vi "testCustomAssertionFailureMessage.vi"() -> ()   [LabVIEW 2019, in "AssertionTest.lvlib" / "ErrorMessageContainsString.lvlib"]
uses:
  ErrorMessageContainsString.lvlib
  Assertion/Assertion.lvlib
  AssertionTest.lvlib
panel:
  out "error out":errorcluster
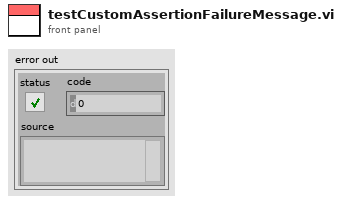
[diagram p1: front panel]
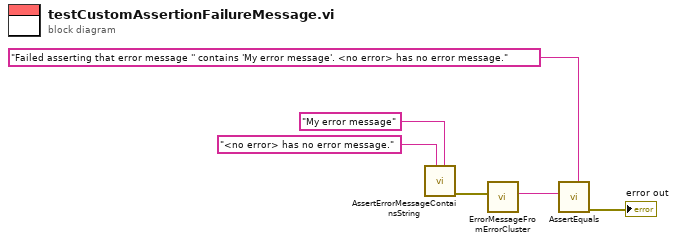
[diagram p0: block diagram]
diagram:
  n1 = call "AssertErrorMessageContainsString.vi"("Expected"="My error message", "Message (\"\")"="<no error> has no error message." ("Message (\"\")")) -> ("error out"=w3:errorcluster)  [unwired: 9 in]
  n2 = call "ErrorMessageFromErrorCluster.vi"("Error"=w3) -> ("Error Message"=w5:string)  [unwired: 10 in]
  n3 = call "AssertEquals.vi"("Expected"="Failed asserting that error message '' contains 'My error message'. <no error> has no error message." ("Needle"), "Actual"=w5) -> ("error out"=→"error out":errorcluster)  [unwired: 9 in]
